vi "분석기.vi"() -> ()   [LabVIEW 2014]
uses:
  <vilib>/Utility/file.llb/Read From Spreadsheet File (string).vi
panel:
  in  "Name":path
  in  "Save_path":path
  in  "Online_Path":path
  in  "Training_Path":path
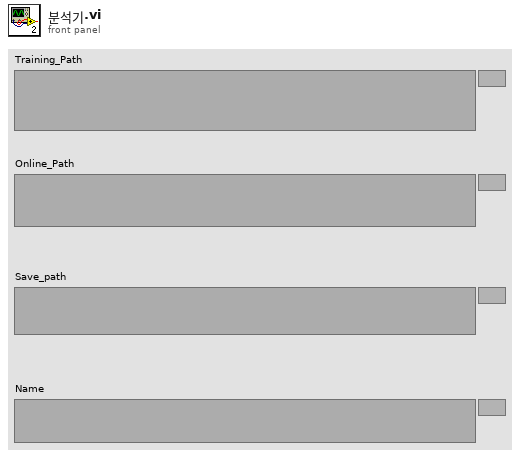
[diagram p1: front panel]
diagram:
  n1 = call-poly <vilib>:"Read From Spreadsheet File.vi"("transpose (no:F)"=TRUE, "file path (dialog if empty)"="Training_Path") -> ("first row"=w10:string[])  [unwired: 5 in, 4 out]
  n2 = call-poly <vilib>:"Read From Spreadsheet File.vi"("transpose (no:F)"=TRUE, "file path (dialog if empty)"="Online_Path") -> ("first row"=w7:string[])  [unwired: 5 in, 4 out]
  n3 = call-poly <vilib>:"Read From Spreadsheet File.vi"("transpose (no:F)"=TRUE, "file path (dialog if empty)"="Save_path") -> ("first row"=w4:string[])  [unwired: 5 in, 4 out]
  n4 = call-poly <vilib>:"Read From Spreadsheet File.vi"("transpose (no:F)"=TRUE, "file path (dialog if empty)"="Name") -> ("first row"=w1:string[])  [unwired: 5 in, 4 out]
  n5 = for {
    tunnel: w10 -> [w14] mode=indexing
    tunnel: w7 -> [w13] mode=indexing
    tunnel: w4 -> [w25] mode=indexing
    tunnel: w1 -> [w15] mode=indexing
    # "1) Training_Path.txt\n2) Online_Path.txt\n3) Save_Path.txt\n4) Name.txt\n를 저장한\ntxt파일을 불러온후 실행하시면 됩니다."
    n6 = Concatenate Strings(w14, "\\ERP_Parameters_of_Target_prior.txt" ("string")) -> (w19:string)
    n7 = Concatenate Strings(w14, "\\ERP_Parameters_of_NonTarget_prior.txt" ("string")) -> (w18:string)
    n8 = String To Path(string=w19) -> (path=w17:path)
    n9 = String To Path(string=w18) -> (path=w16:path)
    n10 = flat-sequence {
      tunnel: [w61] -> w40
      tunnel: [w60] -> w39
      tunnel: [w59] -> w38
      tunnel: [w58] -> w37
      tunnel: [w57] -> w36
      tunnel: [w56] -> w22
      tunnel: w13 -> [w41]
      tunnel: w14 -> [w60]
      tunnel: w25 -> [w56]
      tunnel: w15 -> [w61]
      tunnel: w40 -> [w73]
      tunnel: [w73] -> w35
      tunnel: w39 -> [w75]
      tunnel: [w75] -> w34
      tunnel: w38 -> [w76]
      tunnel: [w76] -> w33
      tunnel: w37 -> [w65]
      tunnel: [w65] -> w32
      tunnel: w36 -> [w64]
      tunnel: [w64] -> w31
      tunnel: [w70] -> w23
      tunnel: w22 -> [w70]
      tunnel: w17 -> [w69]
      tunnel: w16 -> [w68]
      tunnel: [w79] -> w30
      tunnel: [w77] -> w29
      tunnel: [w90] -> w28
      tunnel: [w89] -> w27
      tunnel: [w88] -> w26
      tunnel: [w87] -> w24
      tunnel: w23 -> [w87]
      tunnel: w31 -> [w88]
      tunnel: w32 -> [w89]
      tunnel: w33 -> [w90]
      tunnel: w34 -> [w77]
      tunnel: w35 -> [w79]
      tunnel: w24 -> [w100]
      tunnel: w26 -> [w103]
      tunnel: w27 -> [w101]
      tunnel: w28 -> [w104]
      tunnel: w29 -> [w91]
      tunnel: w30 -> [w102]
      tunnel: w16 -> [w108]
      tunnel: w17 -> [w107]
      frame #0 {
        # "FLDA"
        n11 = Concatenate Strings(w61, "_FLDA" ("string")) -> (w54:string)
        n12 = Concatenate Strings(w60, "\\LDA_Matrix_Value_prior.txt" ("string")) -> (w45:string)
        n13 = Concatenate Strings(w60, "\\Weight_Vector_prior.txt" ("string")) -> (w44:string)
        n14 = Concatenate Strings(w41, "\\Target_order.txt" ("string")) -> (w50:string)
        n15 = Concatenate Strings(w41, "\\mius_flash_order.txt" ("string")) -> (w49:string)
        n16 = Concatenate Strings(w41, "\\Brain.txt" ("string")) -> (w48:string)
        n17 = String To Path(string=w45) -> (path=w43:path)
        n18 = String To Path(string=w44) -> (path=w42:path)
        n19 = String To Path(string=w49) -> (path=w58:path)
        n20 = String To Path(string=w48) -> (path=w57:path)
        n21 = String To Path(string=w50) -> (path=w59:path)
        n22 = call "Offline_Analysis_FLDA_분석기.vi"("LDA_matrix"=w43, "Weight"=w42, "Target_order.txt"=w59, "mius_flash_order"=w58, "Brain"=w57, "피험자이름"=w54, "Save_path"=w56) -> ()  [unwired: 9 in]
      }
      frame #1 {
        # "SVM"
        n23 = Concatenate Strings(w75, "\\LDA_Matrix_Value_SWLDA.txt" ("string")) -> (w67:string)
        n24 = Concatenate Strings(w75, "\\svm_model.model" ("string")) -> (w71:string)
        n25 = Concatenate Strings(w73, "_SVM" ("string")) -> (w72:string)
        n26 = String To Path(string=w67) -> (path=w66:path)
        n27 = call "Offline_Analysis_SVM_분석기.vi"("LDA_matrix"=w66, "Target"=w69, "Nontarget"=w68, "Target_order.txt"=w76, "mius_flash_order"=w65, "Brain"=w64, "svm_model_file"=w71, "피험자이름"=w72, "Save_path"=w70) -> ()  [unwired: 7 in]
      }
      frame #2 {
        # "p-enter = 0.01\np-remove = 0.05"
        # "SWLDA (LDA)"
        n28 = Concatenate Strings(w77, "\\LDA_Matrix_Value_SWLDA.txt") -> (w84:string)
        n29 = Concatenate Strings(w77, "\\Weight_Vector_SWLDA.txt") -> (w83:string)
        n30 = String To Path(string=w84) -> (path=w82:path)
        n31 = String To Path(string=w83) -> (path=w81:path)
        n32 = Concatenate Strings(w79, "_SWLDA" ("string")) -> (w78:string)
        n33 = call "Offline_Analysis__SWLDA_분석기.vi"("LDA_matrix"=w82, "Weight"=w81, "Target_order.txt"=w90, "mius_flash_order"=w89, "Brain"=w88, "피험자이름"=w78, "Save_path"=w87) -> ()  [unwired: 9 in]
      }
      frame #3 {
        # "p-enter = 0.01\np-remove = 0.05"
        # "SWSVM_New (in)"
        n34 = Concatenate Strings(w91, "\\svm_model2.model") -> (w96:string)
        n35 = Concatenate Strings(w91, "\\LDA_Matrix_Value_SWLDA.txt") -> (w94:string)
        n36 = Concatenate Strings(w91, "\\in_SWLDA.txt") -> (w95:string)
        n37 = String To Path(string=w94) -> (path=w98:path)
        n38 = String To Path(string=w95) -> (path=w93:path)
        n39 = Concatenate Strings(w102, "_SWSVM" ("string")) -> (w106:string)
        n40 = call "Offline_Analysis_SWSVM_newSelectionMethod_in_분석기.vi"("LDA_matrix"=w98, "Target"=w107, "Nontarget"=w108, "in_matrix"=w93, "svm_model_file"=w96, "Target_order.txt"=w104, "mius_flash_order"=w101, "Brain"=w103, "피험자이름"=w106, "Save_path"=w100) -> ()  [unwired: 6 in]
      }
    }
  }
